vi "comando.vi"(1 "ANEXO L":string="\u0000", 3 "ANEXO H":string="\u0000", 4 "BYTES IN":u16=255, 5 "LOW":string="\u0000", 6 "HIGH":string="\u0000", 7 "Comando:":u8=1 min=1 max=20 step=1 format="%x", 8 "Equipo Nº":u8) -> (0 "Bytes OUT":u16, 2 "comando":string)   [LabVIEW 2010]
panel:
  out "error out":errorcluster
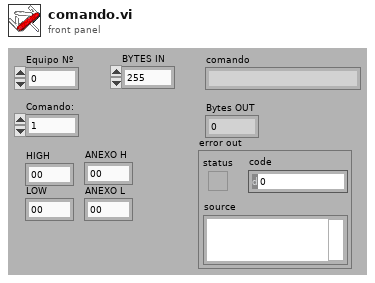
[diagram p1: front panel]
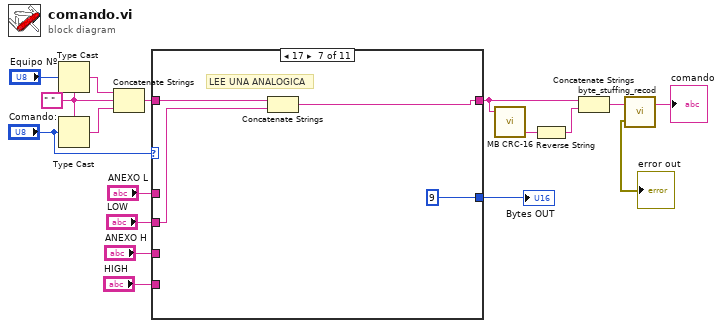
[diagram p0: block diagram]
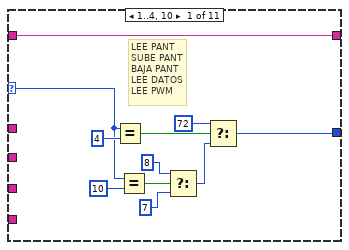
[diagram p2: hidden frame]
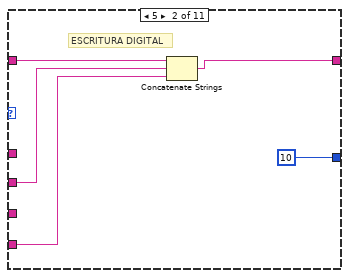
[diagram p3: hidden frame]
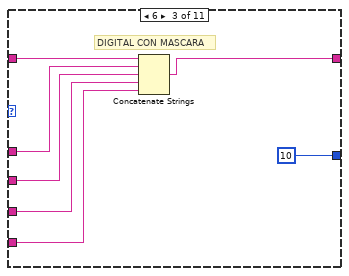
[diagram p4: hidden frame]
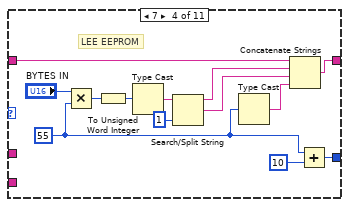
[diagram p5: hidden frame]
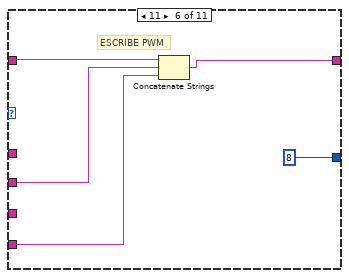
[diagram p7: hidden frame]
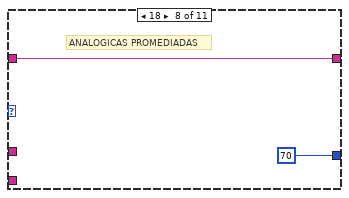
[diagram p8: hidden frame]
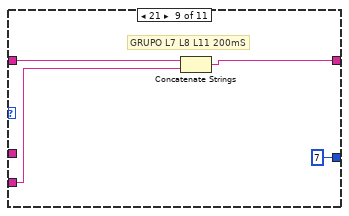
[diagram p9: hidden frame]
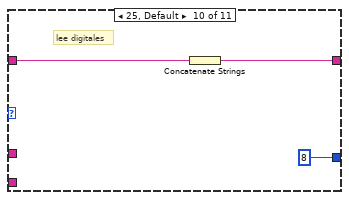
[diagram p10: hidden frame]
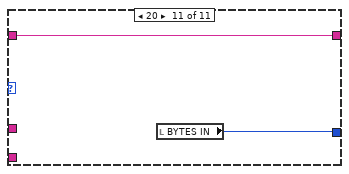
[diagram p11: hidden frame]
diagram:
  w9 = " " ("Lectura 2")
  n1 = Type Cast(type=w9, x="Equipo Nº") -> (*(type *) &x=w13:string)
  n2 = Type Cast(type=w9, x="Comando:") -> (*(type *) &x=w11:string)
  n3 = Concatenate Strings(w13, w9, w11) -> (w10:string)
  n4 = case shown="17" "Comando:" {
    selector: "Comando:" -> [w19 _ _ _ _ _ _ _ _ _ _]
    tunnel: w10 -> [w24 w33 w40 w43 _ w57 w62 w64 w68 w71 w72]
    tunnel: [w24 w32 w39 w42 _ w56 w61 w64 w67 w69 w72] -> w17
    tunnel: [w26 u16 10 ("BYTES READ") u16 10 ("BYTES READ") w53 _ u16 8 ("BYTES IN") u16 9 ("BYTES IN") u16 70 ("BYTES IN") u16 7 ("BYTES IN") u16 8 ("BYTES IN") w73] -> w6
    tunnel: "HIGH" -> [_ w29 w34 _ _ w55 _ _ _ _ _]
    tunnel: "LOW" -> [_ w30 w37 _ _ w54 w59 _ w66 _ _]
    tunnel: "ANEXO L" -> [_ _ w36 _ _ _ _ _ _ _ _]
    tunnel: "ANEXO H" -> [_ _ w35 _ _ _ _ _ _ _ _]
    frame 1..4, 10 {
      # "LEE PANT\nSUBE PANT\nBAJA PANT\nLEE DATOS\nLEE PWM"
      n5 = Equal?(x=w19, y=u8 4) -> (x = y?=w27:bool)
      n6 = Equal?(x=w19, y=u8 10) -> (x = y?=w21:bool)
      n7 = Select(t=u16 8, s=w21, f=u16 7) -> (s? t:f=w18:u16)
      n8 = Select(t=u16 72, s=w27, f=w18) -> (s? t:f=w26:u16)
    }
    frame 5 {
      # "ESCRITURA DIGITAL"
      n9 = Concatenate Strings(w33, w30, w29) -> (w32:string)
    }
    frame 6 {
      # "DIGITAL CON MASCARA"
      n10 = Concatenate Strings(w40, w36, w37, w35, w34) -> (w39:string)
    }
    frame 7 {
      w41 = u16 55 ("y")
      # "LEE EEPROM"
      n11 = Multiply(x="BYTES IN", y=w41) -> (x*y=w46:u16)
      n12 = To Unsigned Word Integer(number=w46) -> (unsigned 16bit integer=w45:u16)
      n13 = Type Cast(x=w45) -> (*(type *) &x=w49:string)  [unwired: 1 in]
      n14 = Search/Split String(string=w49, offset (0)=1) -> (substring before match=w48:string, match + rest of string=w47:string)  [unwired: 1 in, 1 out]
      n15 = Type Cast(x=w41) -> (*(type *) &x=w51:string)  [unwired: 1 in]
      n16 = Concatenate Strings(w43, w48, w47, w51) -> (w42:string)
      n17 = Add(x=w41, y=u16 10) -> (x+y=w53:u16)
    }
    frame 8 {
      # "IMPLENTACION PARTICULAR\nEN VI GRABAR EEPROM"
    }
    frame 11 {
      # "ESCRIBE PWM"
      n18 = Concatenate Strings(w57, w54, w55) -> (w56:string)
    }
    frame 17 {
      # "LEE UNA ANALOGICA"
      n19 = Concatenate Strings(w62, w59) -> (w61:string)
    }
    frame 18 {
      # "ANALOGICAS PROMEDIADAS"
    }
    frame 21 {
      # "GRUPO L7 L8 L11 200mS"
      n20 = Concatenate Strings(w68, w66) -> (w67:string)
    }
    frame 25, Default {
      # "lee digitales"
      n21 = Concatenate Strings(w71) -> (w69:string)
    }
    frame 20 {
      n22 = local read "BYTES IN"() -> (w73:u16)
    }
  }
  "Bytes OUT" <- w6
  n23 = call "MB CRC-16.vi"("String"=w17) -> ("CRC-16"=w15:string)  [unwired: 2 in, 2 out]
  n24 = Reverse String(1:w15) -> (0:w16:string)
  n25 = Concatenate Strings(w17, w16) -> (w3:string)
  n26 = call "byte_stuffing_recod.vi"("String IN"=w3) -> ("String OUT"=→"comando":string, "error out"=→"error out":errorcluster)  [unwired: 1 out]
